vi "功能试验 总圈数.vi"(11 "输入角度":dbl[](array[numeric])) -> (3 "总圈数":dbl)   [LabVIEW 2015, in "Logging.lvlib"]
uses:
  Logging.lvlib
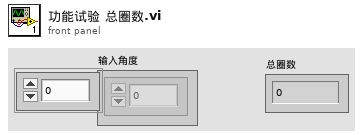
[diagram p1: front panel]
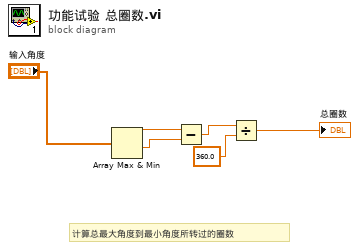
[diagram p0: block diagram]
diagram:
  # "计算总最大角度到最小角度所转过的圈数"
  n1 = Array Max & Min(array="输入角度") -> (max value=w3:dbl, min value=w4:dbl)  [unwired: 2 out]
  n2 = Subtract(x=w3, y=w4) -> (x-y=w5:dbl)
  n3 = Divide(x=w5, y=360.0) -> (x/y=→"总圈数":dbl)
